vi "X509_free.vi"(8 "error in (no error)":errorcluster, 11 "X509-Cert in":refnum<class "X509-Cert.lvclass">) -> (0 "error out":errorcluster)   [LabVIEW 2013, in "SSL_Lib.lvlib" / "X509-Cert.lvclass"]
uses:
  X509-Cert.lvclass
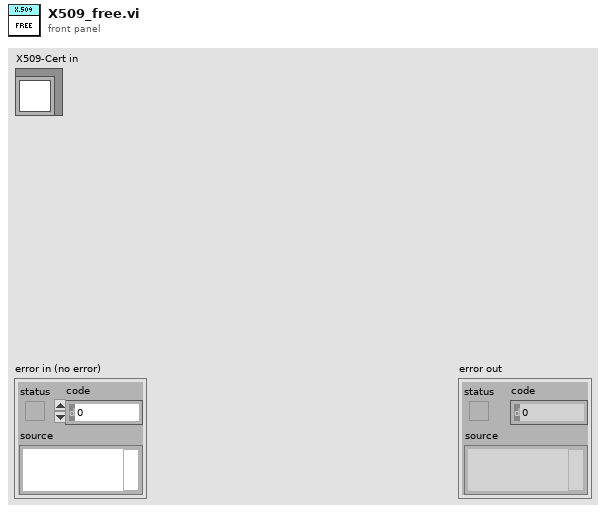
[diagram p1: front panel]
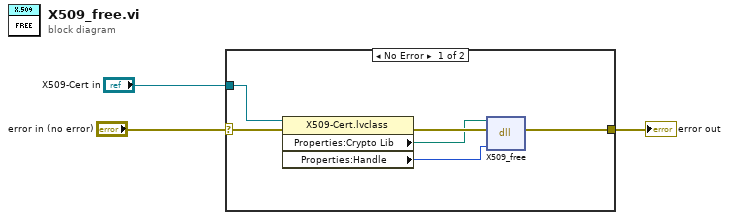
[diagram p0: block diagram]
diagram:
  n1 = case shown="No Error" "error in (no error)" {
    selector: "error in (no error)" -> [w7 w9]
    tunnel: [w6 w9] -> w2
    tunnel: "X509-Cert in" -> [w8 _]
    frame No Error {
      n2 = property class="X509-Cert.lvclass"(reference=w8, error in=w7) -> (error out=w6:errorcluster, "Properties:Crypto Lib"=w4:path, "Properties:Handle"=w5:u64)  [unwired: 1 out]
      n3 = dll-call lib="C:/Program Files (x86)/National Instruments/Shared/nissl/NIlibeay32.dll" fn="X509_free"(path in=w4, error in=w6, "X509"=w5) -> ()  [unwired: 3 in, 2 out]
    }
    frame Error {
    }
  }
  "error out" <- w2
